vi "Configure Measurement (Demodulation - ASK or FSK Analysis).vi"(0 "VISA resource name":refnum<visa-resource-name>, 1 "Measurement Length (20)":dbl=20.0, 5 "Enable Average (F: Disable)":bool, 9 "Average Count (10)":dbl=10.0, 11 "error in (no error)":errorcluster) -> (4 "VISA resource name out":refnum<visa-resource-name>, 15 "error out":errorcluster)   [LabVIEW 2022 SP3, in "Agilent N934X Series.lvlib"]
doc: "Configures the analysis setting for ASK or FSK demodulation of Demodulation Option.\n\nNote:\nThis VI is only applicable for N9321C, N9322C, N9323C, N9324C models"
uses:
  <instrlib>/Agilent N934X Series/Agilent N934X Series.lvlib
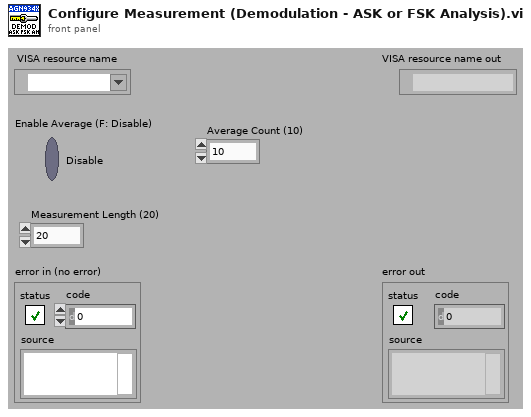
[diagram p1: front panel]
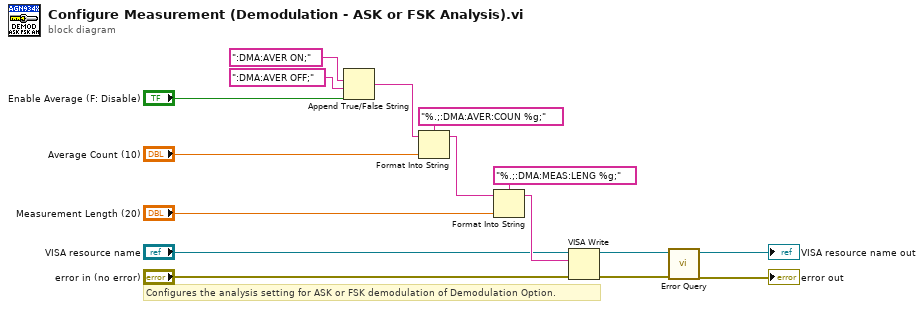
[diagram p0: block diagram]
diagram:
  # "Configures the analysis setting for ASK or FSK demodulation of Demodulation Option."
  n1 = Append True/False String(1:"Enable Average (F: Disable)", 2:":DMA:AVER OFF;", 3:":DMA:AVER ON;") -> (0:w13:string)  [unwired: 1 in]
  n2 = Format Into String(format string="%.;:DMA:AVER:COUN %g;", initial string=w13, "Average Count (10)") -> (resulting string=w10:string)  [unwired: 1 in, 1 out]
  n3 = Format Into String(format string="%.;:DMA:MEAS:LENG %g;", initial string=w10, "Measurement Length (20)") -> (resulting string=w7:string)  [unwired: 1 in, 1 out]
  n4 = VISA Write(VISA resource name="VISA resource name", write buffer=w7, error in (no error)="error in (no error)") -> (VISA resource name out=w4:refnum<visa-resource-name>, error out=w3:errorcluster)  [unwired: 1 out]
  n5 = call <instrlib>:"Error Query.vi"("error in (no error)"=w3, "VISA resource name"=w4) -> ("error out"=→"error out":errorcluster, "VISA resource name out"=→"VISA resource name out":refnum<visa-resource-name>)  [unwired: 6 in, 2 out]
